vi "Page_Dialog_Write.vi"(6 "ctlReferences":T1, 8 "error in (no error)":errorcluster, 11 "Class in":refnum<class "IB_MSI.lvclass">) -> (0 "error out":errorcluster, 3 "Class out":refnum<class "IB_MSI.lvclass">)   [LabVIEW 2020, in "IB_MSI.lvclass"]
uses:
  <vilib>/AppBuilder/IB_Classes/MSI/IB_MSI.lvclass
  <resource>/Framework/Providers/Builds/Installer/Pages/controls/IB_UI_Page_Dialog_Info_References.ctl
  <resource>/Framework/Providers/Builds/Installer/CDK_sTypeDef_Languages.ctl
  <resource>/Framework/Providers/Common/provcom_BrowseProjectFile2.ctl
  <vilib>/AppBuilder/IB_Classes/MSI/IB_MSI.lvclass/IB_MSI.ctl
  <vilib>/AppBuilder/IB_Classes/Installer/Installer.lvclass
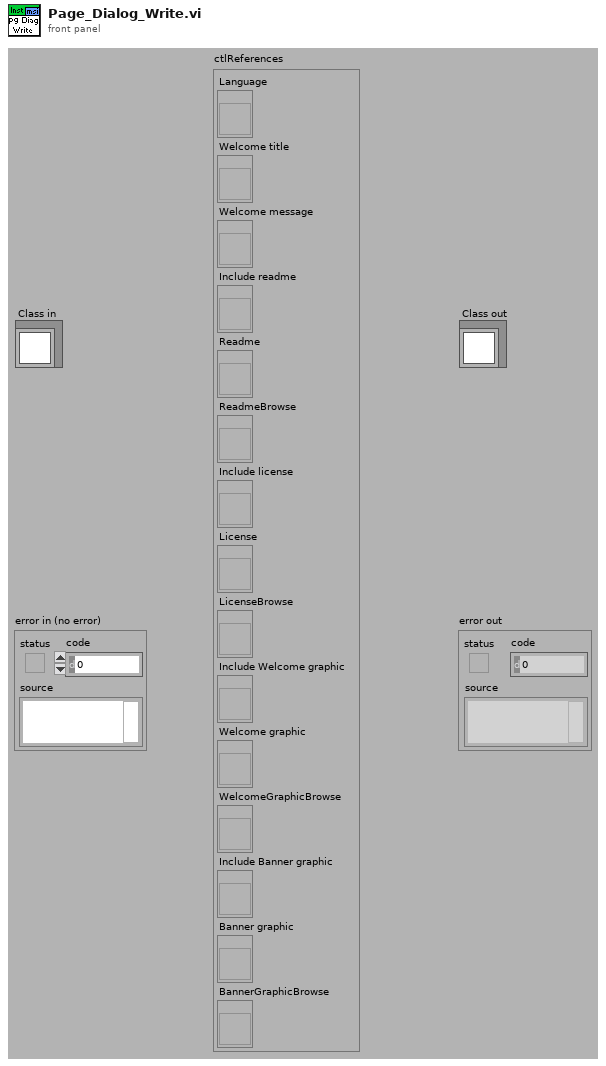
[diagram p1: front panel]
types:
  T1 = typedef "IB_UI_Page_Dialog_Info_References.ctl" = cluster{"Language":refnum<vi>, "Welcome title":refnum<vi>, "Welcome message":refnum<vi>, "Include readme":refnum<vi>, "Readme":refnum<vi>, "ReadmeBrowse":refnum<vi>, "Include license":refnum<vi>, "License":refnum<vi>, "LicenseBrowse":refnum<vi>, "Include Welcome graphic":refnum<vi>, "Welcome graphic":refnum<vi>, "WelcomeGraphicBrowse":refnum<vi>, "Include Banner graphic":refnum<vi>, "Banner graphic":refnum<vi>, "BannerGraphicBrowse":refnum<vi>}
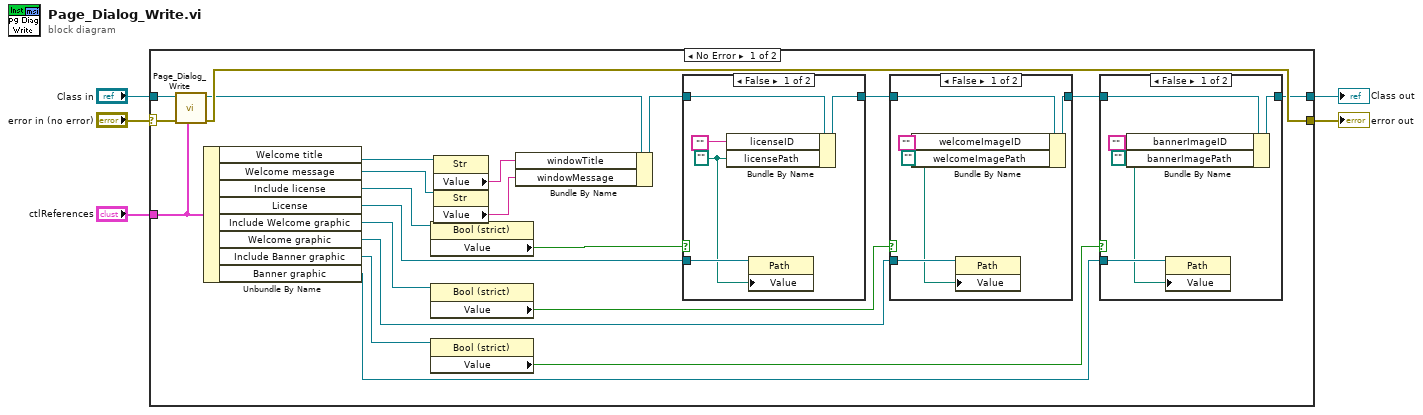
[diagram p0: block diagram]
diagram:
  n1 = case shown="No Error" "error in (no error)" {
    selector: "error in (no error)" -> [w25 w47]
    tunnel: [w24 w47] -> w4
    tunnel: [w12 w46] -> w2
    tunnel: "Class in" -> [w26 w46]
    tunnel: "ctlReferences" -> [w23 _]
    frame No Error {
      n2 = call-parent "Page_Dialog_Write.vi"("ctlReferences"=w23, "error in (no error)"=w25, "Class in"=w26) -> ("error out"=w24:errorcluster, "Class out"=w22:refnum<class "IB_MSI.lvclass">)  [unwired: 7 out]
      n3 = Unbundle By Name(w23) -> ("Welcome title"=w27:refnum<vi>, "Welcome message"=w20:refnum<vi>, "Include license"=w19:refnum<vi>, "License"=w15:refnum<vi>, "Include Welcome graphic"=w11:refnum<vi>, "Welcome graphic"=w9:refnum<vi>, "Include Banner graphic"=w10:refnum<vi>, "Banner graphic"=w6:refnum<vi>)
      n4 = property class="Bool (strict)"(reference=w19) -> ("Value"=w16:bool)  [unwired: 1 in, 2 out]
      n5 = property class="Bool (strict)"(reference=w11) -> ("Value"=w8:bool)  [unwired: 1 in, 2 out]
      n6 = property class="Bool (strict)"(reference=w10) -> ("Value"=w7:bool)  [unwired: 1 in, 2 out]
      n7 = property class="Str"(reference=w27) -> ("Value"=w21:string)  [unwired: 1 in, 2 out]
      n8 = property class="Str"(reference=w20) -> ("Value"=w18:string)  [unwired: 1 in, 2 out]
      n9 = Bundle By Name(cluster=w22, "windowTitle"=w21, "windowMessage"=w18) -> (w17:refnum<class "IB_MSI.lvclass">)
      n10 = case shown="False" w16 {
        tunnel: [w43 w45] -> w14
        tunnel: w17 -> [w44 w45]
        tunnel: w15 -> [w41 _]
        frame False {
          w40 = path ""
          n11 = Bundle By Name(cluster=w44, "licenseID"="", "licensePath"=w40) -> (w43:refnum<class "IB_MSI.lvclass">)
          n12 = property class="Path"(reference=w41, "Value"=w40) -> ()  [unwired: 1 in, 2 out]
        }
        frame True {
        }
      }
      n13 = case shown="False" w8 {
        tunnel: [w37 w39] -> w13
        tunnel: w14 -> [w38 w39]
        tunnel: w9 -> [w35 _]
        frame False {
          w34 = path ""
          n14 = Bundle By Name(cluster=w38, "welcomeImageID"="", "welcomeImagePath"=w34) -> (w37:refnum<class "IB_MSI.lvclass">)
          n15 = property class="Path"(reference=w35, "Value"=w34) -> ()  [unwired: 1 in, 2 out]
        }
        frame True {
        }
      }
      n16 = case shown="False" w7 {
        tunnel: [w31 w33] -> w12
        tunnel: w13 -> [w32 w33]
        tunnel: w6 -> [w29 _]
        frame False {
          w28 = path ""
          n17 = Bundle By Name(cluster=w32, "bannerImageID"="", "bannerImagePath"=w28) -> (w31:refnum<class "IB_MSI.lvclass">)
          n18 = property class="Path"(reference=w29, "Value"=w28) -> ()  [unwired: 1 in, 2 out]
        }
        frame True {
        }
      }
    }
    frame Error {
    }
  }
  "error out" <- w4
  "Class out" <- w2
